vi "Begin.vi"(8 "error in":errorcluster) -> (0 "error out":errorcluster)   [LabVIEW 2014]
doc: "Called before other user functions, this VI is expected to open initial I/O refnums, load in file data, and do all program initialization. Notice that the <B>error out</B> terminal is simply used for data flow. Wiring it to other structures or subVIs ensures that this VI runs first."
uses:
  <vilib>/Rock Robotics/SystemInterfaces/DIO/FPGA_DIOPWMChannel.ctl
  <vilib>/Rock Robotics/WPI/SafetyOutput/WPI_SafetyOutputConfigMenu.ctl
  <vilib>/Rock Robotics/WPI/DriverStation/WPI_DriverStationRobotMode2.ctl
  <vilib>/Rock Robotics/WPI/Joystick/WPI_JoystickDeviceEnum.ctl
  <vilib>/Rock Robotics/SystemInterfaces/DIO/FPGA_DIOChannel.ctl
  <vilib>/Rock Robotics/SystemInterfaces/Typedef/FPGA_TypedefDigitalModule.ctl
  <vilib>/Rock Robotics/WPI/RobotDrive/WPI_RobotDriveOpen2MotorWithVictorSP.vi
  Robot Global Data.vi
  <vilib>/Rock Robotics/Network Tables/SD Write String Array.vi
  <vilib>/Rock Robotics/WPI/Switch/WPI_SwitchOpenLimit.vi
  <vilib>/Rock Robotics/WPI/Counter/WPI_CounterDigitalInputToDigitalSource.vi
  <vilib>/Rock Robotics/WPI/MotorControl/WPI_MotorControlOpen VictorSP.vi
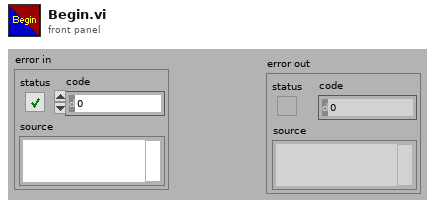
[diagram p1: front panel]
types:
  T1 = typedef "FPGA_TypedefDigitalModule.ctl" = enum16{"Controller 1"}
  T2 = typedef "FPGA_DIOPWMChannel.ctl" = enum8{"PWM 0", "PWM 1", "PWM 2", "PWM 3", "PWM 4", "PWM 5", "PWM 6", "PWM 7", "PWM 8", "PWM 9", "PWM MXP 0", "PWM MXP 1", "PWM MXP 2", "PWM MXP 3", "PWM MXP 4", "PWM MXP 5", "PWM MXP 6", "PWM MXP 7", "PWM MXP 8", "PWM MXP 9", "Invalid"}
  T3 = typedef "FPGA_DIOChannel.ctl" = enum8{"DIO 0", "DIO 1", "DIO 2", "DIO 3", "DIO 4", "DIO 5", "DIO 6", "DIO 7", "DIO 8", "DIO 9", "DIO MXP 0", "DIO MXP 1", "DIO MXP 2", "DIO MXP 3", "DIO MXP 4", "DIO MXP 5", "DIO MXP 6", "DIO MXP 7", "DIO MXP 8", "DIO MXP 9", "DIO MXP 10", "DIO MXP 11", "DIO MXP 12", "DIO MXP 13", "DIO MXP 14", "DIO MXP 15", "Invalid"}
  T4 = typedef "WPI_JoystickDeviceEnum.ctl" = enum16{"USB 0", "USB 1", "USB 2", "USB 3", "USB 4", "USB 5"}
  T5 = typedef "WPI_DriverStationRobotMode2.ctl" = enum16{"Autonomous Disabled", "Autonomous Enabled", "Teleop Disabled", "Teleop Enabled", "Disconnected", "Finish", "Test Disabled", "Test Enabled", "Emergency Stopped"}
  T6 = typedef "WPI_SafetyOutputConfigMenu.ctl" = enum16{"Enable", "Disable"}
  T7 = typedef "WPI_RobotDriveDevRef.ctl" = cluster{"DevStatus":errorcluster, "Motors[]":T8[], "Square Inputs":bool, "Max Output":dbl}
  T8 = typedef "WPI_MotorControlDeviceRef.ctl" = cluster{"DeviceStatus":errorcluster, "Type":T9, "PWM":cluster{"Controller":T1, "PWM Channel":T2, "DeadBand":T10}, "CAN":cluster{"Device Number":u8, "Control Mode":T11, "Semaphore":T12, "Max Vout":dbl, "TalonSRX Control Mode":T13}, "Invert":bool, "TransformRef":T14, "InvTransformRef":T14}
  T9 = typedef "WPI_MotorControlType.ctl" = enum16{"PWM", "CAN", "CANTalonSRX"}
  T10 = typedef "WPI_PWMDeadband.ctl" = cluster{"Name":string, "maxPositivePwm":i32, "minPositivePwm":i32, "centerPwm":i32, "maxNegativePwm":i32, "minNegativePwm":i32, "angularRange":u16}
  T11 = typedef "WPI_CANJaguar_ControlMode.ctl" = enum8{"Percent VBus", "Current", "Speed", "Position", "Voltage"}
  T12 = typedef "Semaphore RefNum" = refnum<k1>
  T13 = typedef "WPI_CANTalonSRX_APIControlMode.ctl" = enum8{"Percent VBus", "Speed", "Position", "Slave", "Unchanged / Invalid"}
  T14 = typedef "WPI_PWMTransform_ConPane.ctl" = refnum<vi>
  T15 = typedef "WPI_DigitalInputDevRef.ctl" = cluster{"DevStatus":errorcluster, "DIO Channel":T3, "Controller":T1}
  T16 = typedef "FPGA_CounterEncoderSourceConvertionLVSourceType.ctl" = cluster{"DevStatus":errorcluster, "AnalogTriggerMode?":bool, "DigitalMode":cluster{"Controller":T1, "DIO Channel":T17}, "AnalogTriggerMode":cluster{"AnalogTriggerIndex":T18, "OutputType":T19}}
  T17 = typedef "FPGA_DIODigitalSourceChannel.ctl" = enum8{"DIO 0", "DIO 1", "DIO 2", "DIO 3", "DIO 4", "DIO 5", "DIO 6", "DIO 7", "DIO 8", "DIO 9", "DIO MXP 0", "DIO MXP 1", "DIO MXP 2", "DIO MXP 3", "DIO MXP 4", "DIO MXP 5", "DIO MXP 6", "DIO MXP 7", "DIO MXP 8", "DIO MXP 9", "DIO MXP 10", "DIO MXP 11", "DIO MXP 12", "DIO MXP 13", "DIO MXP 14", "DIO MXP 15", "Disabled"}
  T18 = typedef "FPGA_AnalogTriggerIndex.ctl" = enum8{"Trig 0", "Trig 1", "Trig 2", "Trig 3", "Trig 4", "Trig 5", "Trig 6", "Trig 7", "Invalid"}
  T19 = typedef "FPGA_AnalogTriggerOutType.ctl" = enum16{"InWindow", "TriggerState", "Rising", "Falling"}
  T20 = typedef "WPI_SwitchDevRef.ctl" = cluster{"DevStatus":errorcluster, "DIO Channel":T3, "Controller":T1, "CntIndex":T21, "Normally Closed":bool}
  T21 = typedef "FPGA_CounterCtrSystemIndex.ctl" = enum8{"Ctr 0", "Ctr 1", "Ctr 2", "Ctr 3", "Ctr 4", "Ctr 5", "Ctr 6", "Ctr 7", "Invalid"}
  T22 = typedef "WPI_EncoderDevRef.ctl" = cluster{"DevStatus":errorcluster, "EncoderIndex":T23, "CounterIndex":T21, "DistancePerCount":dbl, "Decoding Type":T24}
  T23 = typedef "FPGA_EncoderIdx.ctl" = enum8{"Enc 0", "Enc 1", "Enc 2", "Enc 3", "Enc 4", "Enc 5", "Enc 6", "Enc 7", "Invalid"}
  T24 = typedef "WPI_EncoderType.ctl" = enum16{"1x", "2x", "4x"}
  T25 = typedef "WPI_JoystickDevRef.ctl" = cluster{"Device":T4}
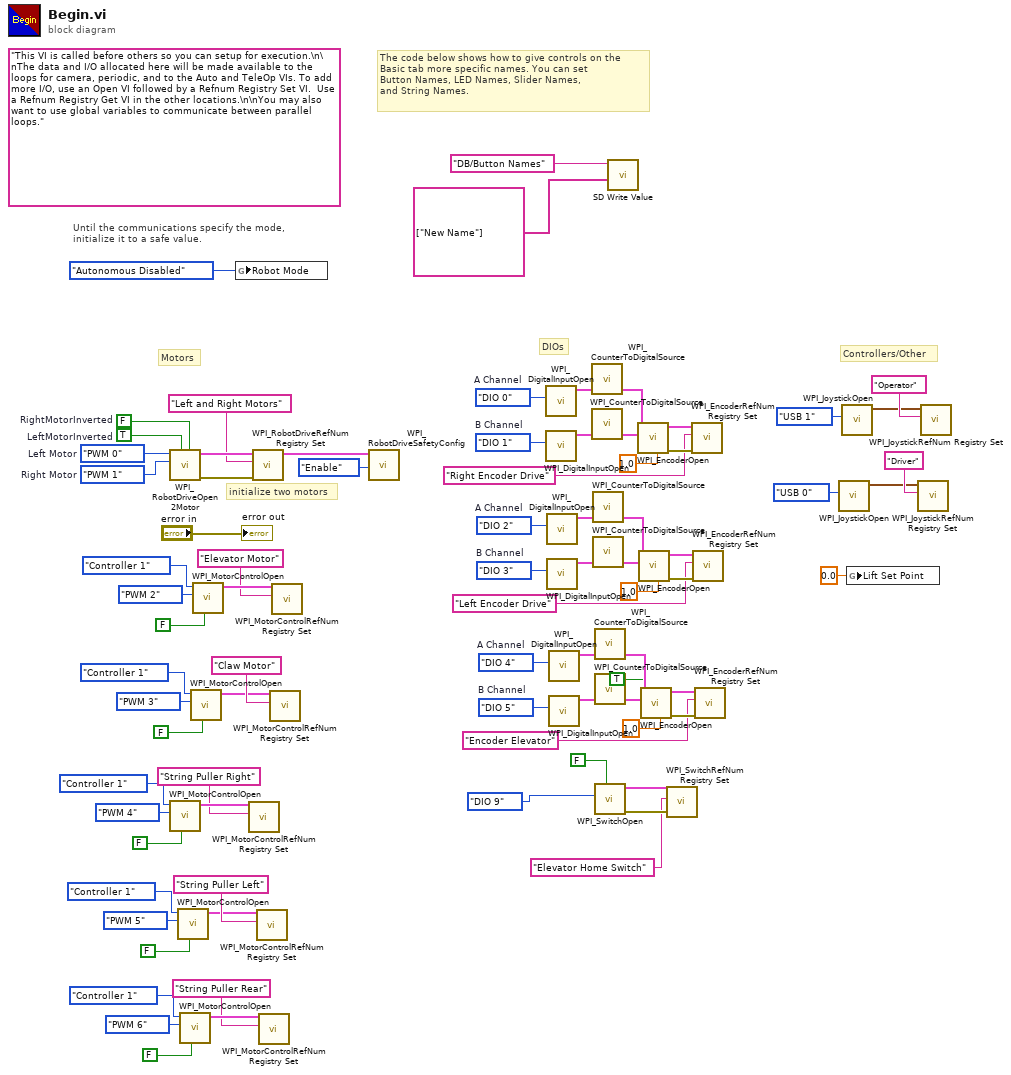
[diagram p0: block diagram]
diagram:
  w25 = FPGA_DIOChannel."DIO 3"  # B Channel
  w24 = FPGA_DIOChannel."DIO 2"  # A Channel
  w35 = FPGA_DIOChannel."DIO 1"  # B Channel
  w34 = FPGA_DIOChannel."DIO 0"  # A Channel
  w60 = FPGA_DIOChannel."DIO 5"  # B Channel
  w59 = FPGA_DIOChannel."DIO 4"  # A Channel
  (unwired) "This VI is called before others so you can setup for execution.\n\nThe data and I/O allocated here will be made available to the loops for camera, periodic, and to the Auto and TeleOp VIs. To add more I/O, use an Open VI followed by a Refnum Registry Set VI.  Use a Refnum Registry Get VI in the other locations.\n\nYou may also want to use global variables to communicate between parallel loops."
  w75 = FPGA_DIOPWMChannel."PWM 1"  # Right Motor
  w76 = FPGA_DIOPWMChannel."PWM 0"  # Left Motor
  w80 = TRUE  # LeftMotorInverted
  w81 = FALSE  # RightMotorInverted
  # "Controllers/Other"
  # "DIOs"
  # "Motors"
  # "The code below shows how to give controls on the\nBasic tab more specific names. You can set\nButton Names, LED Names, Slider Names,\nand String Names."
  # "Until the communications specify the mode,\ninitialize it to a safe value."
  # "initialize two motors"
  n1 = call-poly <vilib>:"WPI_RobotDriveOpen2Motor.vi"("Right Motor Inverted"=w81, "Left Motor Inverted"=w80, "Right Motor"=w75, "Left Motor"=w76) -> ("error out"=w77:errorcluster, "RobotDriveDevRef"=w79:T7)  [unwired: 1 in, 5 out]
  n2 = call-poly <vilib>:"WPI_MotorControlOpen.vi"("Invert"=FALSE, "PWM Channel"=FPGA_DIOPWMChannel."PWM 4", "Controller"=FPGA_TypedefDigitalModule."Controller 1") -> ("MotorControlDeviceRef"=w13:T8)  [unwired: 7 in, 1 out]
  n3 = call-poly <vilib>:"WPI_MotorControlOpen.vi"("Invert"=FALSE, "PWM Channel"=FPGA_DIOPWMChannel."PWM 5", "Controller"=FPGA_TypedefDigitalModule."Controller 1") -> ("MotorControlDeviceRef"=w8:T8)  [unwired: 7 in, 1 out]
  n4 = call-poly <vilib>:"WPI_MotorControlOpen.vi"("Invert"=FALSE, "PWM Channel"=FPGA_DIOPWMChannel."PWM 6", "Controller"=FPGA_TypedefDigitalModule."Controller 1") -> ("MotorControlDeviceRef"=w3:T8)  [unwired: 7 in, 1 out]
  n5 = call-poly <vilib>:"WPI_MotorControlOpen.vi"("Invert"=FALSE, "PWM Channel"=FPGA_DIOPWMChannel."PWM 3", "Controller"=FPGA_TypedefDigitalModule."Controller 1") -> ("MotorControlDeviceRef"=w39:T8)  [unwired: 7 in, 1 out]
  n6 = call-poly <vilib>:"WPI_MotorControlOpen.vi"("Invert"=FALSE, "PWM Channel"=FPGA_DIOPWMChannel."PWM 2", "Controller"=FPGA_TypedefDigitalModule."Controller 1") -> ("MotorControlDeviceRef"=w48:T8)  [unwired: 7 in, 1 out]
  n7 = global write "Robot Global Data.vi" "Robot Mode"(WPI_DriverStationRobotMode2."Autonomous Disabled" ("Robot Mode")) -> ()
  n8 = call <vilib>:"WPI_MotorControlRefNum Registry Set.vi"("refnum name"="String Puller Right", "MotorControlDevRef"=w13) -> ()  [unwired: 8 in, 2 out]
  n9 = call <vilib>:"WPI_RobotDriveRefNum Registry Set.vi"("error in (no error)"=w77, "refnum name"="Left and Right Motors", "RobotDriveDevRef"=w79) -> ("RobotDriveDevRef"=w74:T7)  [unwired: 8 out]
  n10 = call <vilib>:"WPI_MotorControlRefNum Registry Set.vi"("refnum name"="String Puller Left", "MotorControlDevRef"=w8) -> ()  [unwired: 8 in, 2 out]
  n11 = call <vilib>:"WPI_MotorControlRefNum Registry Set.vi"("refnum name"="String Puller Rear", "MotorControlDevRef"=w3) -> ()  [unwired: 8 in, 2 out]
  n12 = call <vilib>:"WPI_MotorControlRefNum Registry Set.vi"("refnum name"="Claw Motor", "MotorControlDevRef"=w39) -> ()  [unwired: 8 in, 2 out]
  n13 = call <vilib>:"WPI_MotorControlRefNum Registry Set.vi"("refnum name"="Elevator Motor", "MotorControlDevRef"=w48) -> ()  [unwired: 8 in, 2 out]
  n14 = call <vilib>:"WPI_RobotDriveSafetyConfig.vi"("mode"=WPI_SafetyOutputConfigMenu."Enable", "RobotDriveDevRef"=w74) -> ()  [unwired: 8 in, 2 out]
  n15 = call <vilib>:"WPI_DigitalInputOpen.vi"("DIO Channel"=w34) -> ("DigitalInputDevRef"=w31:T15)  [unwired: 2 in, 8 out]
  n16 = call <vilib>:"WPI_DigitalInputOpen.vi"("DIO Channel"=w35) -> ("DigitalInputDevRef"=w32:T15)  [unwired: 2 in, 8 out]
  n17 = call <vilib>:"WPI_DigitalInputOpen.vi"("DIO Channel"=w24) -> ("DigitalInputDevRef"=w21:T15)  [unwired: 2 in, 8 out]
  n18 = call <vilib>:"WPI_DigitalInputOpen.vi"("DIO Channel"=w25) -> ("DigitalInputDevRef"=w22:T15)  [unwired: 2 in, 8 out]
  n19 = call <vilib>:"WPI_DigitalInputOpen.vi"("DIO Channel"=w59) -> ("DigitalInputDevRef"=w56:T15)  [unwired: 2 in, 8 out]
  n20 = call <vilib>:"WPI_DigitalInputOpen.vi"("DIO Channel"=w60) -> ("DigitalInputDevRef"=w57:T15)  [unwired: 2 in, 8 out]
  n21 = call-poly <vilib>:"WPI_CounterToDigitalSource.vi"("DigitalInputDevRef"=w31) -> ("Digital Source"=w30:T16)  [unwired: 6 out]
  n22 = call-poly <vilib>:"WPI_CounterToDigitalSource.vi"("DigitalInputDevRef"=w32) -> ("Digital Source"=w33:T16)  [unwired: 6 out]
  n23 = call-poly <vilib>:"WPI_CounterToDigitalSource.vi"("DigitalInputDevRef"=w21) -> ("Digital Source"=w20:T16)  [unwired: 6 out]
  n24 = call-poly <vilib>:"WPI_CounterToDigitalSource.vi"("DigitalInputDevRef"=w22) -> ("Digital Source"=w23:T16)  [unwired: 6 out]
  n25 = call-poly <vilib>:"WPI_CounterToDigitalSource.vi"("DigitalInputDevRef"=w56) -> ("Digital Source"=w55:T16)  [unwired: 6 out]
  n26 = call-poly <vilib>:"WPI_CounterToDigitalSource.vi"("DigitalInputDevRef"=w57) -> ("Digital Source"=w58:T16)  [unwired: 6 out]
  n27 = call-poly <vilib>:"WPI_SwitchOpen.vi"("Normally Closed"=FALSE, "DIO Channel"=FPGA_DIOChannel."DIO 9") -> ("error out"=w62:errorcluster, "SwitchDevRef"=w63:T20)  [unwired: 8 in]
  n28 = call-poly <vilib>:"SD Write Value.vi"("String Array"=string[] ["New Name"], "Name"="DB/Button Names") -> ()  [unwired: 8 in, 2 out]
  n29 = call <vilib>:"WPI_EncoderOpen.vi"("DistancePerCount"=1.0, "BSource"=w33, "ASource"=w30) -> ("error out"=w29:errorcluster, "EncoderDevRef"=w28:T22)  [unwired: 5 in, 2 out]
  n30 = call <vilib>:"WPI_EncoderOpen.vi"("DistancePerCount"=1.0, "BSource"=w23, "ASource"=w20) -> ("error out"=w19:errorcluster, "EncoderDevRef"=w18:T22)  [unwired: 5 in, 2 out]
  n31 = call <vilib>:"WPI_EncoderOpen.vi"("DistancePerCount"=1.0, "Invert Direction (False)"=TRUE, "BSource"=w58, "ASource"=w55) -> ("error out"=w54:errorcluster, "EncoderDevRef"=w53:T22)  [unwired: 4 in, 2 out]
  n32 = call <vilib>:"WPI_SwitchRefNum Registry Set.vi"("error in (no error)"=w62, "refnum name"="Elevator Home Switch", "SwitchDevRef"=w63) -> ()  [unwired: 7 in, 2 out]
  n33 = call <vilib>:"WPI_EncoderRefNum Registry Set.vi"("error in (no error)"=w29, "refnum name"="Right Encoder Drive", "EncoderDevRef"=w28) -> ()  [unwired: 7 in, 2 out]
  n34 = call <vilib>:"WPI_EncoderRefNum Registry Set.vi"("error in (no error)"=w19, "refnum name"="Left Encoder Drive", "EncoderDevRef"=w18) -> ()  [unwired: 7 in, 2 out]
  n35 = call <vilib>:"WPI_EncoderRefNum Registry Set.vi"("error in (no error)"=w54, "refnum name"="Encoder Elevator", "EncoderDevRef"=w53) -> ()  [unwired: 7 in, 2 out]
  n36 = call <vilib>:"WPI_JoystickOpen.vi"("JoystickDevice"=WPI_JoystickDeviceEnum."USB 0") -> ("JoystickDevRef"=w70:T25)  [unwired: 10 in]
  n37 = call <vilib>:"WPI_JoystickOpen.vi"("JoystickDevice"=WPI_JoystickDeviceEnum."USB 1") -> ("JoystickDevRef"=w45:T25)  [unwired: 10 in]
  n38 = global write "Robot Global Data.vi" "Lift Set Point"(0.0 ("Lift Set Point")) -> ()
  n39 = call <vilib>:"WPI_JoystickRefNum Registry Set.vi"("refnum name"="Driver", "JoystickDevRef"=w70) -> ()  [unwired: 8 in, 2 out]
  n40 = call <vilib>:"WPI_JoystickRefNum Registry Set.vi"("refnum name"="Operator", "JoystickDevRef"=w45) -> ()  [unwired: 8 in, 2 out]
  "error out" <- "error in"
